vi "FA_Central Process.vi"() -> ()   [LabVIEW 2014, in "FA_Central Process.lvlib"]
uses:
  FA_Central Process.lvlib
  Shared Code/AMC/VI Source/CentralProcessMessaging/Flock_Shared_CentralProcessMessaging.lvlib
  Shared Code/AMC/VI Source/Flock_Shared_Messaging.lvlib
  Shared Code/AMC/VI Source/ProcessList.ctl
  Shared Code/AMC/VI Source/LocalProcessMessaging/Flock_Shared_LocalProcessMessaging.lvlib
  Shared Code/AMC/VI Source/Error Handling/Flock_ErrorHandling.lvlib
  FA_AgentConfig API/source/VI Source/FA_AgentConfig.lvlib
  StateValue.ctl
panel:
  in  "Stop Button":bool
  in  "Dev":bool
  out "Status":string
  out "Idle Status":string
  # "Stop Button implementation is just for the template."
  # "Set as True if running Central Process in development environment"
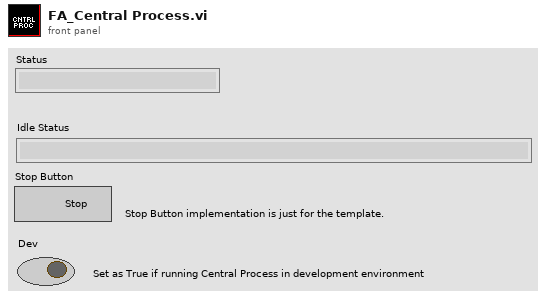
[diagram p1: front panel]
types:
  T1 = typedef "FA_Central Process.lvlib/StateValue.ctl" = enum16{"Available", "Working"}
  T2 = typedef "Flock_Shared_Messaging.lvlib/ProcessList.ctl" = string
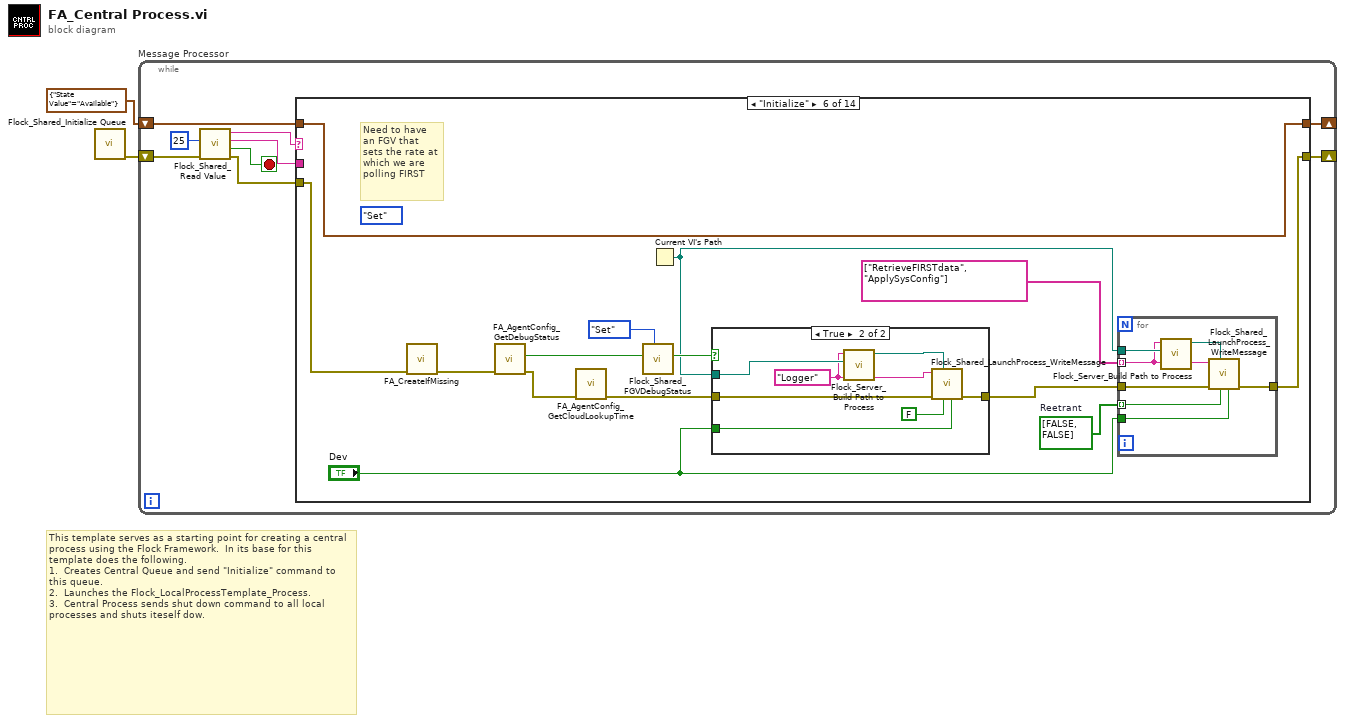
[diagram p0: block diagram]
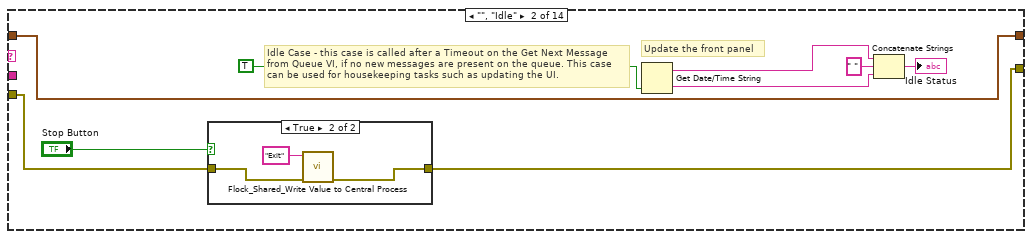
[diagram p3: hidden frame]
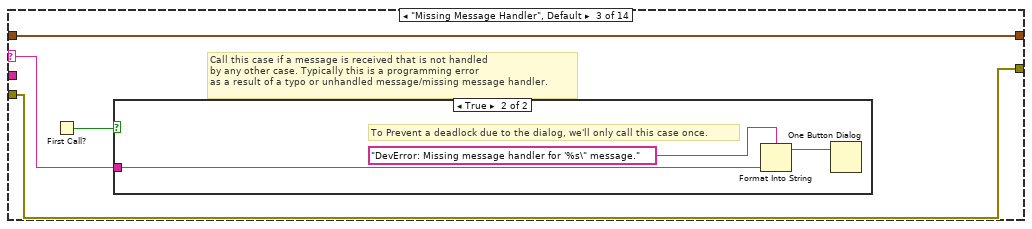
[diagram p5: hidden frame]
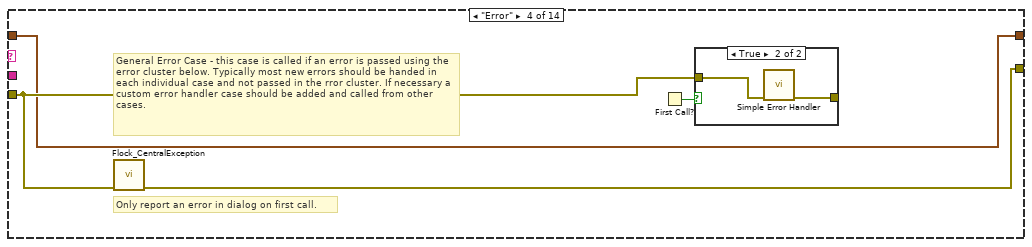
[diagram p7: hidden frame]
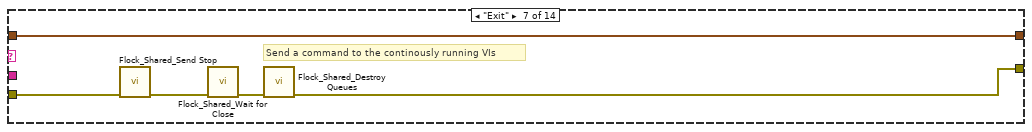
[diagram p11: hidden frame]
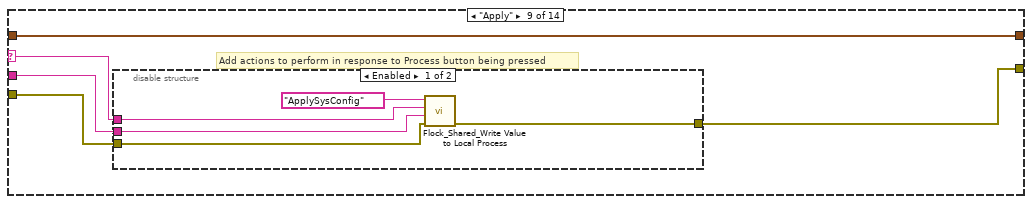
[diagram p13: hidden frame]
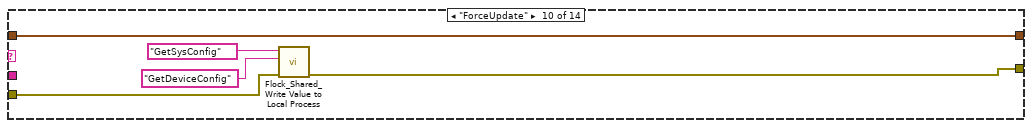
[diagram p15: hidden frame]
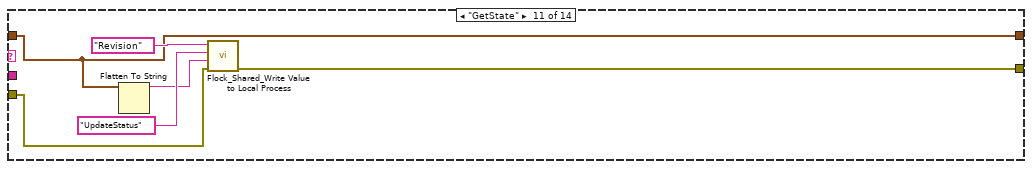
[diagram p16: hidden frame]
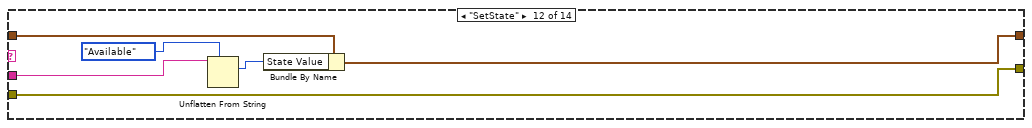
[diagram p17: hidden frame]
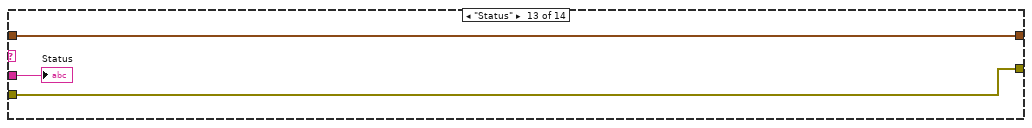
[diagram p18: hidden frame]
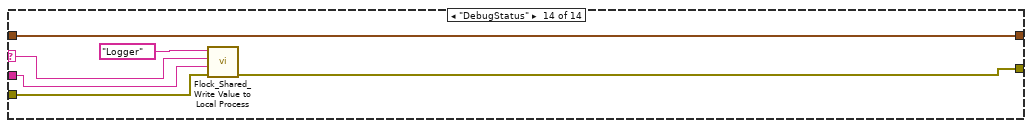
[diagram p19: hidden frame]
diagram:
  # "This template serves as a starting point for creating a central process using the Flock Framework.  In its base for this template does the following.\n1.  Creates Central Queue and send \"Initialize\" command to this queue.\n2.  Launches the Flock_LocalProcessTemplate_Process.\n3.  Central Process sends shut down command to all local processes and shuts iteself dow."
  n1 = call "Flock_Shared_Initialize Queue.vi"() -> ("error out"=w2:errorcluster)  [unwired: 11 in]
  n2 = while "Message Processor" {
    shift-left: w2 -> [w10]
    shift-right: [w11] -> _
    shift-right: [w3] -> _
    shift-left: cluster{"State Value":T1} {"State Value"=enum."Available"} ("StateInformation") -> [w4]
    stop <- w8 stop-if-true
    n3 = call "Flock_Shared_Read Value.vi"("error in (no error)"=w10, "timeout (1ms)"=25) -> ("error out"=w9:errorcluster, "Exit Process"=w8:bool, "Message Value"=w6:string, "Message Name"=w7:string)  [unwired: 6 in]
    n4 = case shown="\"Initialize\"" w7 {
      selector: w7 -> [_ _ w29 _ _ _ _ _ w81 _ _ _ _ w111]
      tunnel: w9 -> [w13 w16 w30 w36 w42 w45 w75 w78 w83 w92 w97 w105 w107 w113]
      tunnel: [w13 w15 w30 w35 w42 w51 w76 w78 w80 w91 w96 w105 w107 w112] -> w11
      tunnel: w6 -> [_ _ _ _ _ _ _ _ w82 _ _ w104 w108 w110]
      tunnel: w4 -> [w12 w14 w27 w34 w41 w46 w72 w77 w79 w93 w95 w101 w106 w109]
      tunnel: [w12 w14 w27 w34 w41 w46 w72 w77 w79 w93 w95 w100 w106 w109] -> w3
      frame "---------- Framework Operations ----------" {
        # "Dummy case to add a seperator in the Case Structure menu"
      }
      frame "", "Idle" {
        # "Update the front panel"
        # "Idle Case - this case is called after a Timeout on the Get Next Message from Queue VI, if no new messages are present on the queue. This case can be used for housekeeping tasks such as updating the UI."
        n5 = case shown="True" "Stop Button" {
          tunnel: w16 -> [w23 w25]
          tunnel: [w23 w24] -> w15
          frame False {
          }
          frame True {
            n6 = call "Flock_Shared_Write Value to Central Process.vi"("error in (no error)"=w25, "Message Name"="Exit") -> ("error out"=w24:errorcluster)  [unwired: 9 in]
          }
        }
        n7 = Get Date/Time String(want seconds? (F)=TRUE) -> (date string=w22:string, time string=w21:string)  [unwired: 2 out]
        n8 = Concatenate Strings(w22, " " ("string"), w21) -> (→"Idle Status":string)
      }
      frame "Missing Message Handler", Default {
        # "Call this case if a message is received that is not handled \nby any other case. Typically this is a programming error\nas a result of a typo or unhandled message/missing message handler."
        n9 = First Call?() -> (First Call?: T/F=w28:bool)
        n10 = case shown="True" w28 {
          tunnel: w29 -> [_ w33]
          frame False {
          }
          frame True {
            # "To Prevent a deadlock due to the dialog, we'll only call this case once."
            n11 = Format Into String(format string="DevError: Missing message handler for '%s\" message." ("message"), w33) -> (resulting string=w31:string)  [unwired: 2 in, 1 out]
            n12 = One Button Dialog(message=w31) -> ()  [unwired: 2 out]
          }
        }
      }
      frame "Error" {
        # "Only report an error in dialog on first call."
        # "General Error Case - this case is called if an error is passed using the error cluster below. Typically most new errors should be handed in each individual case and not passed in the rror cluster. If necessary a custom error handler case should be added and called from other cases."
        n13 = call "Flock_CentralException.vi"("Error In"=w36) -> ("Error Out"=w35:errorcluster)  [unwired: 10 in]
        n14 = First Call?() -> (First Call?: T/F=w37:bool)
        n15 = case shown="True" w37 {
          tunnel: w36 -> [w38 w40]
          tunnel: [w38 w39] -> _
          frame False {
          }
          frame True {
            n16 = call <vilib>:"Simple Error Handler.vi"("error in (no error)"=w40) -> ("error out"=w39:errorcluster)  [unwired: 1 in, 7 out]
          }
        }
      }
      frame "---------- Generic Operations ----------" {
        # "Dummy case to add a seperator in the Case Structure menu"
      }
      frame "Initialize" {
        w49 = bool[] [FALSE, FALSE]  # Reetrant
        (unwired) enum16{"Get", "Set"}."Set" ("State")
        # "Need to have an FGV that sets the rate at which we are polling FIRST"
        n17 = call "FA_CreateIfMissing.vi"("Error In"=w45) -> ("Error Out"=w44:errorcluster)  [unwired: 10 in]
        n18 = call "FA_AgentConfig_GetDebugStatus.vi"("Error In"=w44) -> ("Error Out"=w50:errorcluster, "DebugStatus"=w56:bool)  [unwired: 9 in]
        n19 = call "FA_AgentConfig_GetCloudLookupTime.vi"("Error In"=w50) -> ("Error Out"=w47:errorcluster)  [unwired: 9 in, 1 out]
        n20 = call "Flock_Shared_FGVDebugStatus.vi"("State"=enum16{"Get", "Set"}."Set", "DebugBoolean"=w56) -> ("Debug Boolean"=w54:bool)  [unwired: 9 in]
        n21 = Current VI's Path() -> (path=w53:path)
        n22 = case shown="True" w54 {
          tunnel: w53 -> [_ w71]
          tunnel: [w64 w68] -> w52
          tunnel: "Dev" -> [_ w66]
          tunnel: w47 -> [w64 w65]
          frame False {
          }
          frame True {
            w69 = T2 "Logger" ("Process")
            n23 = call "Flock_Server_Build Path to Process.vi"("path"=w71, "Process"=w69) -> ("Local Process Path"=w70:path)  [unwired: 9 in]
            n24 = call "Flock_Shared_LaunchProcess_WriteMessage.vi"("Show Front Panel?"=w66, "Reentrant?"=FALSE, "VI Path"=w70, "error in (no error)"=w65, "Process List"=w69) -> ("error out"=w68:errorcluster)  [unwired: 6 in]
          }
        }
        n25 = for {
          tunnel: w49 -> [w62] mode=indexing
          tunnel: w53 -> [w61]
          tunnel: w52 -> [w60]
          tunnel: [w59] -> w51
          tunnel: "Dev" -> [w58]
          tunnel: T2[] ["RetrieveFIRSTdata", "ApplySysConfig"] -> [w57] mode=indexing
          n26 = call "Flock_Server_Build Path to Process.vi"("path"=w61, "Process"=w57) -> ("Local Process Path"=w63:path)  [unwired: 9 in]
          n27 = call "Flock_Shared_LaunchProcess_WriteMessage.vi"("Show Front Panel?"=w58, "Reentrant?"=w62, "VI Path"=w63, "error in (no error)"=w60, "Process List"=w57) -> ("error out"=w59:errorcluster)  [unwired: 6 in]
        }
      }
      frame "Exit" {
        # "Send a command to the continously running VIs"
        n28 = call "Flock_Shared_Send Stop.vi"("error in (no error)"=w75) -> ("error out"=w74:errorcluster)  [unwired: 10 in]
        n29 = call "Flock_Shared_Wait for Close.vi"("error in (no error)"=w74) -> ("error out"=w73:errorcluster)  [unwired: 10 in]
        n30 = call "Flock_Shared_Destroy Queues.vi"("error in (no error)"=w73) -> ("error out"=w76:errorcluster)  [unwired: 10 in]
      }
      frame "---------- Application Operations ----------" {
        # "Dummy case to add a seperator in the Case Structure menu"
      }
      frame "Apply" {
        # "Add actions to perform in response to Process button being pressed"
        n31 = disable-structure shown="Enabled" {
          disable-tunnel: w83 -> [w88 _]
          disable-tunnel: w82 -> [w87 _]
          disable-tunnel: w81 -> [w86 _]
          disable-tunnel: [w85 _] -> w80
          frame Enabled {
            n32 = call "Flock_Shared_Write Value to Local Process.vi"("error in (no error)"=w88, "Message Value"=w87, "Message Name"=w86, "Process List"=T2 "ApplySysConfig" ("Process")) -> ("error out"=w85:errorcluster)  [unwired: 7 in]
          }
          frame Disabled {
          }
        }
      }
      frame "ForceUpdate" {
        n33 = call "Flock_Shared_Write Value to Local Process.vi"("error in (no error)"=w92, "Message Name"="GetDeviceConfig", "Process List"=T2 "GetSysConfig") -> ("error out"=w91:errorcluster)  [unwired: 8 in]
      }
      frame "GetState" {
        n34 = Flatten To String(anything=w95) -> (data string=w94:string)  [unwired: 3 in, 2 out]
        n35 = call "Flock_Shared_Write Value to Local Process.vi"("error in (no error)"=w97, "Message Value"=w94, "Message Name"="UpdateStatus", "Process List"=T2 "Revision") -> ("error out"=w96:errorcluster)  [unwired: 7 in]
      }
      frame "SetState" {
        n36 = Unflatten From String(type=StateValue."Available" ("State Value"), binary string=w104) -> (value=w102:T1)  [unwired: 3 in, 2 out]
        n37 = Bundle By Name(cluster=w101, "State Value"=w102) -> (w100:cluster{"State Value":T1})
      }
      frame "Status" {
        "Status" <- w108
      }
      frame "DebugStatus" {
        n38 = call "Flock_Shared_Write Value to Local Process.vi"("error in (no error)"=w113, "Message Value"=w110, "Message Name"=w111, "Process List"=T2 "Logger" ("Process")) -> ("error out"=w112:errorcluster)  [unwired: 7 in]
      }
    }
  }
